vi "pp_saveStimParam.vi"(0 "Total Trials":i32=2 min=2, 4 "Stims 1":dbl[][](array[numeric]), 5 "Stims 2":dbl[][](array[numeric]), 9 "error in (no error)":errorcluster) -> (10 "Path":path, 13 "error out":errorcluster)   [LabVIEW 2013]
uses:
  <vilib>/Utility/xml.llb/Write to XML File(array).vi
panel:
  in  "Trial Randomization":enum32{"50% exactly", "Radio Selection 2"}(radio)
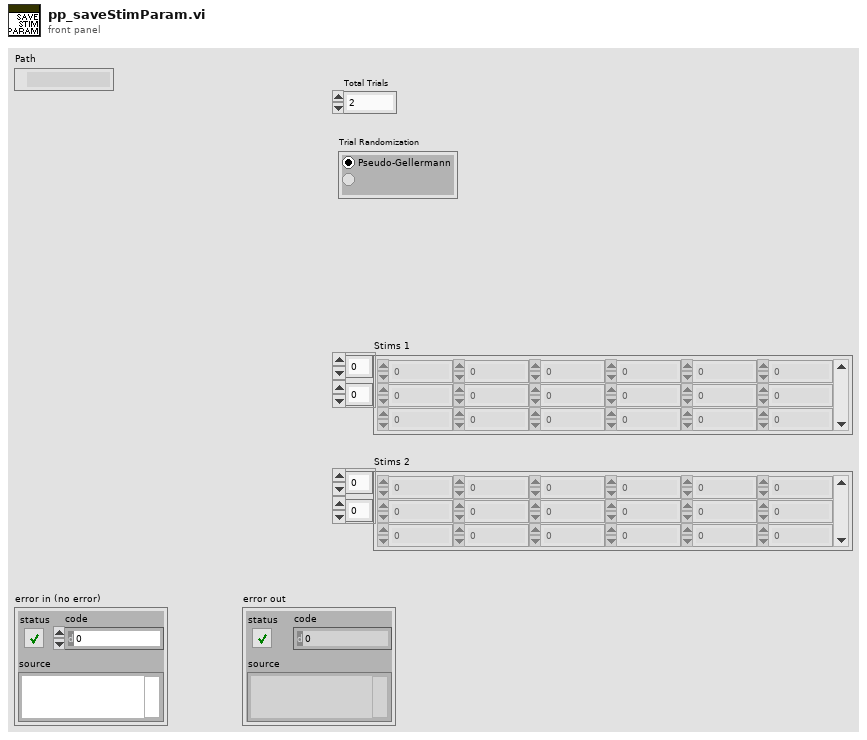
[diagram p1: front panel]
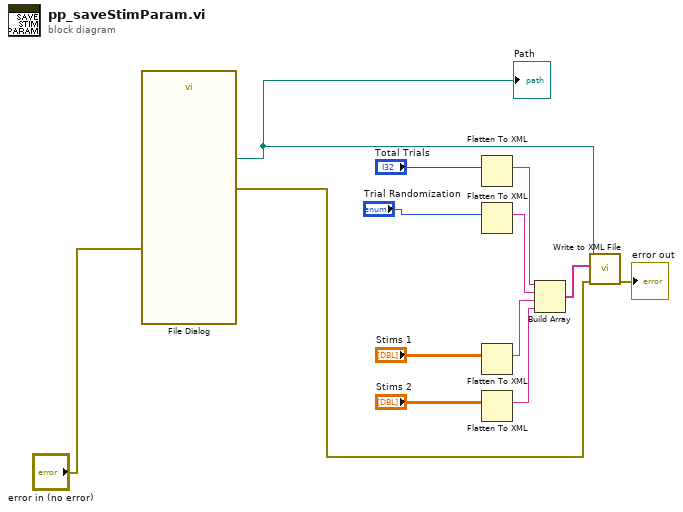
[diagram p0: block diagram]
diagram:
  n1 = call "File Dialog"("error in"="error in (no error)") -> ("selected path"=w12:path, "error out"=w10:errorcluster)  [unwired: 11 in, 2 out]
  "Path" <- w12
  n2 = Flatten To XML(anything="Total Trials") -> (xml string=w6:string)
  n3 = Flatten To XML(anything="Trial Randomization") -> (xml string=w5:string)
  n4 = Flatten To XML(anything="Stims 1") -> (xml string=w2:string)
  n5 = Flatten To XML(anything="Stims 2") -> (xml string=w1:string)
  n6 = Build Array(w6, w5, w2, w1) -> (w4:string[])
  n7 = call-poly <vilib>:"Write to XML File.vi"("error in (no error)"=w10, "XML Input"=w4, "XML File Path"=w12) -> ("error out"=→"error out":errorcluster)  [unwired: 6 in, 2 out]
